vi "Global Variable Logic.vi"() -> ()   [LabVIEW 2020]
uses:
  Global 1.vi
panel:
  in  "stop":bool
  out "String 2":string
  in  "String":string
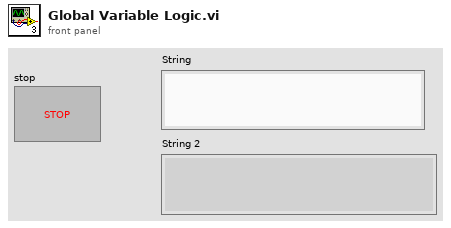
[diagram p1: front panel]
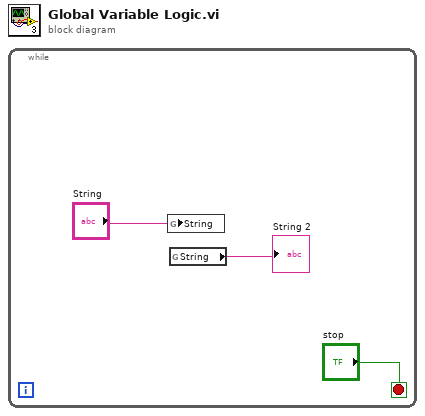
[diagram p0: block diagram]
diagram:
  n1 = while {
    stop <- "stop" stop-if-true
    n2 = global write "Global 1.vi" "String"("String") -> ()
    n3 = global read "Global 1.vi" "String"() -> (→"String 2":string)
  }
